vi "CreateSQLstring.vi"(10 "string":string, 11 "Array":string[](array[string])) -> (3 "String":string)   [LabVIEW 2017, in "Server.lvlib" / "Oracle.lvlib"]
uses:
  Oracle.lvlib
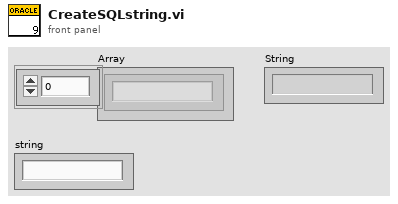
[diagram p1: front panel]
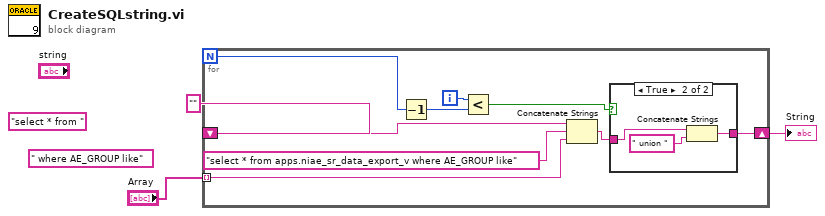
[diagram p0: block diagram]
diagram:
  (unwired) " where AE_GROUP like" ("string")
  (unwired) "select * from " ("SQL query")
  n1 = for {
    N -> [w12]
    tunnel: "Array" -> [w4] mode=indexing
    shift-right: [w7] -> w3
    shift-left: "" -> [w6]
    i -> [w11]
    n2 = Decrement(x=w12) -> (x-1=w10:i32)
    n3 = Less?(x=w11, y=w10) -> (x < y?=w9:bool)
    n4 = Concatenate Strings(w6, "select * from apps.niae_sr_data_export_v where AE_GROUP like" ("SQL query"), w4) -> (w8:string)
    n5 = case shown="True" w9 {
      tunnel: w8 -> [w13 w16]
      tunnel: [w13 w14] -> w7
      frame False {
      }
      frame True {
        n6 = Concatenate Strings(w16, " union " ("string")) -> (w14:string)
      }
    }
  }
  "String" <- w3
